vi "Obtain Request Events.vi"(8 "error in":errorcluster, 10 "Create New? (F)":bool) -> (0 "error out":errorcluster, 2 "Host Interpreter Request Events":T1)   [LabVIEW 2021, in "Host Interpreter.lvlib"]
doc: "This VI Obtains/Creates the Requests events that will be used for other modules to communicate with the module that owns this VI. These Requests events will be accessed only via Public API methods for this module.\n\n<b>NOTE</b>: The contents of this VI are automatically generated and modified by the <b>Tools > DQMH Consortium > DQMH</b> utilities. Consider using those utilities instead of making your own modifications to this VI.\n_____\nBased on DQMH Dev Tools: Project Template 7.1.2.1547."
uses:
  Host Interpreter.lvlib
  Request Events--cluster.ctl
  Stop Argument--cluster.ctl
  Show Panel Argument--cluster.ctl
  Hide Panel Argument--cluster.ctl
  Get Module Execution Status Argument--cluster.ctl
  Show Diagram Argument--cluster.ctl
  Connect to Target Argument--cluster.ctl
  Get Config Argument--cluster.ctl
  Open UDP Argument--cluster.ctl
  Start Reading MSGs Argument--cluster.ctl
  Send Message to Target Argument--cluster.ctl
  Libraries/UDP Comms/UDP Message--cluster.ctl
  Request Connections to Target Argument--cluster.ctl
  Close UDP Argument--cluster.ctl
  Update Polling Time Argument--cluster.ctl
  Disconnect from Target Argument--cluster.ctl
  Connected to Target Argument--cluster.ctl
  Disconnected from Target Argument--cluster.ctl
  Libraries/UDP Comms/UDP Comms.lvlib
panel:
  # "NOTE: The contents of this VI are automatically generated and modified by the Tools > DQMH Consortium > DQMH utilities. Consider using those utilities instead of making your own modifications to this VI."
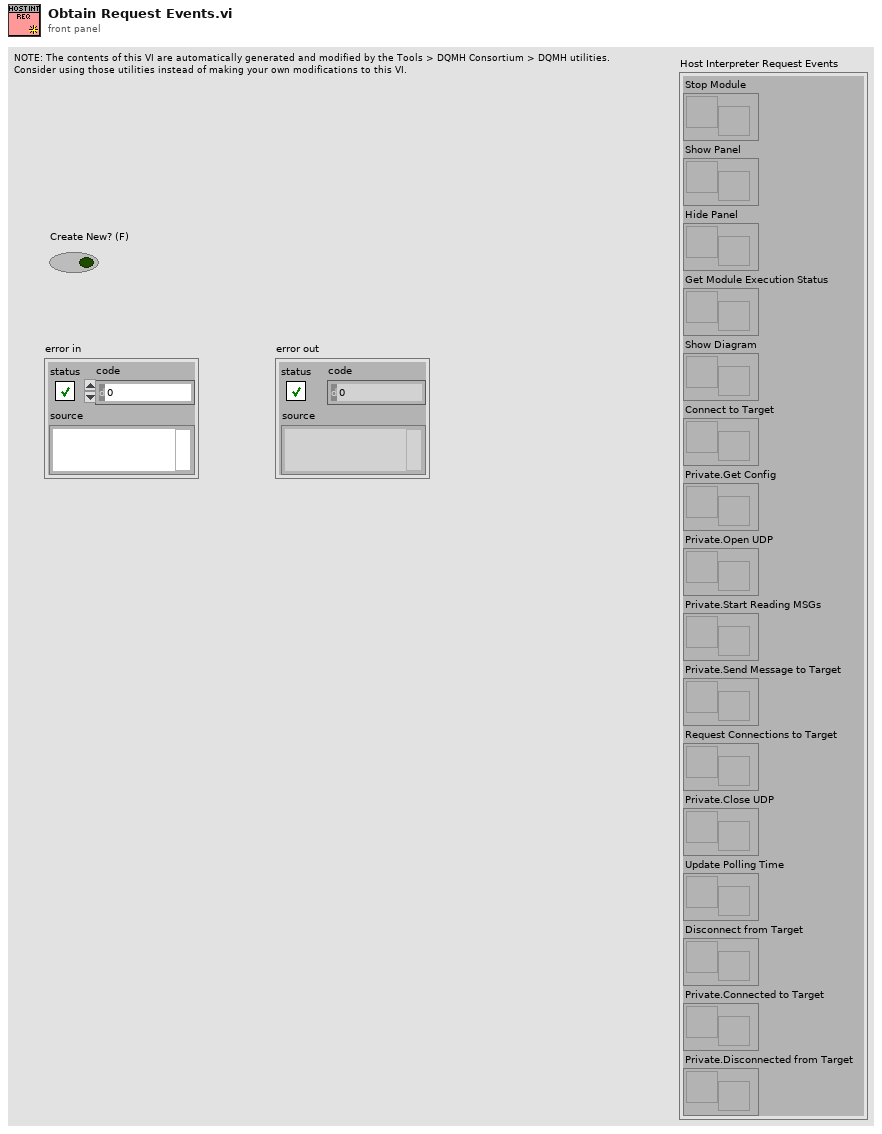
[diagram p1: front panel]
types:
  T1 = typedef "Host Interpreter.lvlib/Request Events--cluster.ctl" = cluster{"Stop Module":refnum<user-event>, "Show Panel":refnum<user-event>, "Hide Panel":refnum<user-event>, "Get Module Execution Status":refnum<user-event>, "Show Diagram":refnum<user-event>, "Connect to Target":refnum<user-event>, "Private.Get Config":refnum<user-event>, "Private.Open UDP":refnum<user-event>, "Private.Start Reading MSGs":refnum<user-event>, "Private.Send Message to Target":refnum<user-event>, "Request Connections to Target":refnum<user-event>, "Private.Close UDP":refnum<user-event>, "Update Polling Time":refnum<user-event>, "Disconnect from Target":refnum<user-event>, "Private.Connected to Target":refnum<user-event>, "Private.Disconnected from Target":refnum<user-event>}
  T2 = typedef "Host Interpreter.lvlib/Disconnected from Target Argument--cluster.ctl" = cluster{"Boolean":bool}
  T3 = typedef "Host Interpreter.lvlib/Connected to Target Argument--cluster.ctl" = cluster{"Boolean":bool}
  T4 = typedef "Host Interpreter.lvlib/Disconnect from Target Argument--cluster.ctl" = cluster{"Boolean":bool}
  T5 = typedef "Host Interpreter.lvlib/Update Polling Time Argument--cluster.ctl" = cluster{"Poling Time":i32}
  T6 = typedef "Host Interpreter.lvlib/Close UDP Argument--cluster.ctl" = cluster{"Boolean":bool}
  T7 = typedef "Host Interpreter.lvlib/Request Connections to Target Argument--cluster.ctl" = cluster{"Boolean":bool}
  T8 = typedef "Host Interpreter.lvlib/Send Message to Target Argument--cluster.ctl" = cluster{"First Message?":bool, "UDP Message":T9}
  T9 = typedef "UDP Comms.lvlib/UDP Message--cluster.ctl" = cluster{"Command":string, "Data":variant}
  T10 = typedef "Host Interpreter.lvlib/Start Reading MSGs Argument--cluster.ctl" = cluster{"Polling Rate (ms)":i32, "Host UDP connection ref":refnum<k16>, "Target IP":string, "Target UDP Listening Port":u16}
  T11 = typedef "Host Interpreter.lvlib/Open UDP Argument--cluster.ctl" = cluster{"Boolean":bool}
  T12 = typedef "Host Interpreter.lvlib/Get Config Argument--cluster.ctl" = cluster{"Boolean":bool}
  T13 = typedef "Host Interpreter.lvlib/Connect to Target Argument--cluster.ctl" = cluster{"Boolean":bool}
  T14 = typedef "Host Interpreter.lvlib/Hide Panel Argument--cluster.ctl" = cluster{"Hide Panel?":bool}
  T15 = typedef "Host Interpreter.lvlib/Show Panel Argument--cluster.ctl" = cluster{"Show Panel?":bool}
  T16 = typedef "Host Interpreter.lvlib/Show Diagram Argument--cluster.ctl" = cluster{"Debug?":bool}
  T17 = typedef "Host Interpreter.lvlib/Get Module Execution Status Argument--cluster.ctl" = cluster{"Running?":bool}
  T18 = typedef "Host Interpreter.lvlib/Stop Argument--cluster.ctl" = cluster{"Origin":string, "Exit via Stop Module Req?":bool, "Wait for Module to stop?":bool}
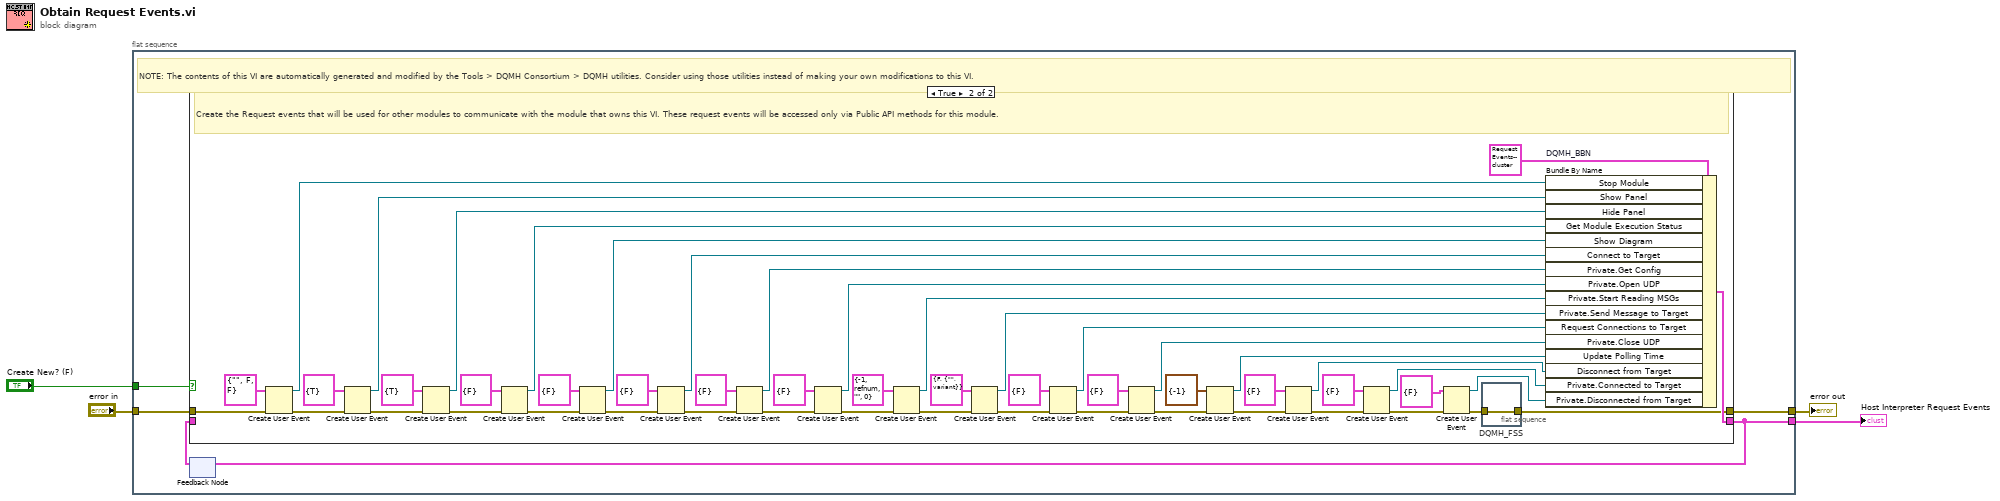
[diagram p0: block diagram]
diagram:
  n1 = flat-sequence {
    tunnel: [w9] -> w4
    tunnel: "error in" -> [w8]
    tunnel: [w6] -> w2
    tunnel: "Create New? (F)" -> [w5]
    frame #0 {
      # "NOTE: The contents of this VI are automatically generated and modified by the Tools > DQMH Consortium > DQMH utilities. Consider using those utilities instead of making your own modifications to this VI."
      n2 = feedback #1() -> (w7:T1)  [unwired: 1 in]
      n3 = case shown="True" w5 {
        tunnel: [w10 w53] -> w9
        tunnel: w8 -> [w10 w63]
        tunnel: [w11 w60] -> w6
        tunnel: w7 -> [w11 _]
        frame False {
          # "Obtain the Request events that were created in a previous call to this VI."
        }
        frame True {
          # "Create the Request events that will be used for other modules to communicate with the module that owns this VI. These request events will be accessed only via Public API methods for this module."
          n4 = Create User Event(user event datatype=T18 {"Origin"="", "Exit via Stop Module Req?"=FALSE, "Wait for Module to stop?"=FALSE} ("Stop Argument"), error in=w63) -> (user event=w61:refnum<user-event>, error out=w58:errorcluster)
          n5 = Create User Event(user event datatype=T15 {"Show Panel?"=TRUE} ("Show Panel Argument"), error in=w58) -> (user event=w57:refnum<user-event>, error out=w56:errorcluster)
          n6 = Create User Event(user event datatype=T14 {"Hide Panel?"=TRUE} ("Hide Panel Argument"), error in=w56) -> (user event=w55:refnum<user-event>, error out=w54:errorcluster)
          n7 = Create User Event(user event datatype=T17 {"Running?"=FALSE} ("Get Module Execution Status Argument"), error in=w54) -> (user event=w51:refnum<user-event>, error out=w52:errorcluster)
          n8 = Create User Event(user event datatype=T16 {"Debug?"=FALSE} ("Show Diagram Argument"), error in=w52) -> (user event=w48:refnum<user-event>, error out=w49:errorcluster)
          n9 = Create User Event(user event datatype=T13 {"Boolean"=FALSE} ("Connect to Target Argument"), error in=w49) -> (user event=w43:refnum<user-event>, error out=w44:errorcluster)
          n10 = Create User Event(user event datatype=T12 {"Boolean"=FALSE} ("Get Host Config Argument"), error in=w44) -> (user event=w40:refnum<user-event>, error out=w41:errorcluster)
          n11 = Create User Event(user event datatype=T11 {"Boolean"=FALSE} ("Open UDP Argument"), error in=w41) -> (user event=w37:refnum<user-event>, error out=w38:errorcluster)
          n12 = Create User Event(user event datatype=T10 {"Polling Rate (ms)"=-1, "Host UDP connection ref"=refnum, "Target IP"="", "Target UDP Listening Port"=0} ("Start Reading MSGs Argument"), error in=w38) -> (user event=w34:refnum<user-event>, error out=w35:errorcluster)
          n13 = Create User Event(user event datatype=T8 {"First Message?"=FALSE, "UDP Message"={"Command"="", "Data"=variant}} ("Send Message to Target Argument"), error in=w35) -> (user event=w31:refnum<user-event>, error out=w32:errorcluster)
          n14 = Create User Event(user event datatype=T7 {"Boolean"=FALSE} ("Request Connections to Target Argument"), error in=w32) -> (user event=w28:refnum<user-event>, error out=w29:errorcluster)
          n15 = Create User Event(user event datatype=T6 {"Boolean"=FALSE} ("Close UDP Argument"), error in=w29) -> (user event=w25:refnum<user-event>, error out=w26:errorcluster)
          n16 = Create User Event(user event datatype=T5 {"Poling Time"=-1} ("Update Polling Time Argument"), error in=w26) -> (user event=w22:refnum<user-event>, error out=w23:errorcluster)
          n17 = Create User Event(user event datatype=T4 {"Boolean"=FALSE} ("Disconnect from Target Argument"), error in=w23) -> (user event=w19:refnum<user-event>, error out=w20:errorcluster)
          n18 = Create User Event(user event datatype=T3 {"Boolean"=FALSE} ("Connected to Target Argument"), error in=w20) -> (user event=w16:refnum<user-event>, error out=w17:errorcluster)
          n19 = Create User Event(user event datatype=T2 {"Boolean"=FALSE} ("Disconnected from Target Argument"), error in=w17) -> (user event=w13:refnum<user-event>, error out=w14:errorcluster)
          n20 = flat-sequence "DQMH_FSS" {
            tunnel: w14 -> [w64]
            tunnel: [w64] -> w53
            frame #0 {
            }
          }
          n21 = Bundle By Name "DQMH_BBN"(cluster=T1 {"Stop Module"=refnum, "Show Panel"=refnum, "Hide Panel"=refnum, "Get Module Execution Status"=refnum, "Show Diagram"=refnum, "Connect to Target"=refnum, "Private.Get Config"=refnum, "Private.Open UDP"=refnum, "Private.Start Reading MSGs"=refnum, "Private.Send Message to Target"=refnum, "Request Connections to Target"=refnum, "Private.Close UDP"=refnum, "Update Polling Time"=refnum, "Disconnect from Target"=refnum, "Private.Connected to Target"=refnum, "Private.Disconnected from Target"=refnum} ("output cluster"), "Stop Module"=w61, "Show Panel"=w57, "Hide Panel"=w55, "Get Module Execution Status"=w51, "Show Diagram"=w48, "Connect to Target"=w43, "Private.Get Config"=w40, "Private.Open UDP"=w37, "Private.Start Reading MSGs"=w34, "Private.Send Message to Target"=w31, "Request Connections to Target"=w28, "Private.Close UDP"=w25, "Update Polling Time"=w22, "Disconnect from Target"=w19, "Private.Connected to Target"=w16, "Private.Disconnected from Target"=w13) -> (w60:T1)
        }
      }
      n22 = feedback-in #1(w6) -> ()
    }
  }
  "Host Interpreter Request Events" <- w2
  "error out" <- w4
